vi "Shell Crossflow Area.vi"(9 "Dctl (m)":dbl, 10 "MHX Tube Pitch (m)":dbl, 11 "MHX Tube Diameter (m)":dbl) -> (3 "Shell Crossflow Area (m^2)":dbl)   [LabVIEW 2019]
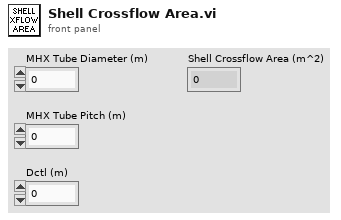
[diagram p1: front panel]
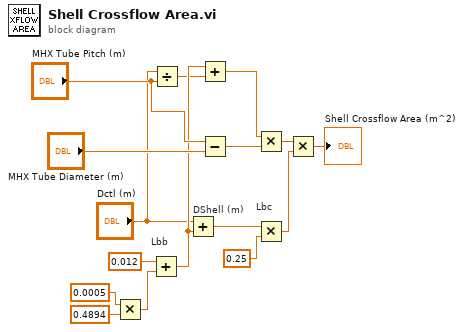
[diagram p0: block diagram]
diagram:
  n1 = Multiply(x=0.0005, y=0.4894) -> (x*y=w3:dbl)
  n2 = Add "Lbb"(x=0.012, y=w3) -> (x+y=w10:dbl)
  n3 = Divide(x="Dctl (m)", y="MHX Tube Pitch (m)") -> (x/y=w9:dbl)
  n4 = Add "DShell (m)"(x="Dctl (m)", y=w10) -> (x+y=w6:dbl)
  n5 = Add(x=w10, y=w9) -> (x+y=w11:dbl)
  n6 = Subtract(x="MHX Tube Pitch (m)", y="MHX Tube Diameter (m)") -> (x-y=w14:dbl)
  n7 = Multiply(x=w11, y=w14) -> (x*y=w15:dbl)
  n8 = Multiply "Lbc"(x=w6, y=0.25) -> (x*y=w7:dbl)
  n9 = Multiply(x=w15, y=w7) -> (x*y=→"Shell Crossflow Area (m^2)":dbl)
